vi "Write to session log.vi"(1 "Session string":string="#Running Custom Tests") -> ()   [LabVIEW 2019]
uses:
  Board_Global_Var.vi
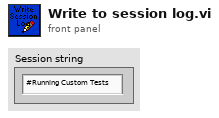
[diagram p1: front panel]
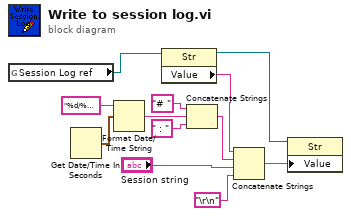
[diagram p0: block diagram]
diagram:
  n1 = global read "Board_Global_Var.vi" "Session Log ref"() -> (w1:refnum<vi>)
  n2 = Get Date/Time In Seconds() -> (seconds since 1Jan1904=w7:timestamp)
  n3 = Format Date/Time String(time format string (%c)="%d/%m/%y_%H:%M:%S", seconds (now)=w7) -> (date/time string=w9:string)  [unwired: 1 in]
  n4 = property on="Property Node" class="Str"(reference=w1) -> (reference out=w2:refnum<vi>, "Value"=w3:string)  [unwired: 1 in, 1 out]
  n5 = Concatenate Strings("# " ("string"), w9, " : " ("string")) -> (w12:string)
  n6 = Concatenate Strings(w3, w12, "Session string", "\r\n") -> (w4:string)
  n7 = property on="Property Node" class="Str"(reference=w2, "Value"=w4) -> ()  [unwired: 1 in, 2 out]
